vi "aggregator - v - real - interp.vi"(8 "number":dbl, 10 "init?":bool, 11 "requested size":i32=20) -> (0 "slope":dbl, 1 "interp average":dbl, 2 "mean":dbl, 3 "Array":dbl[](array[numeric]))   [LabVIEW 2018]
uses:
  agregator -- action.ctl
  linear interpolation - real.vi
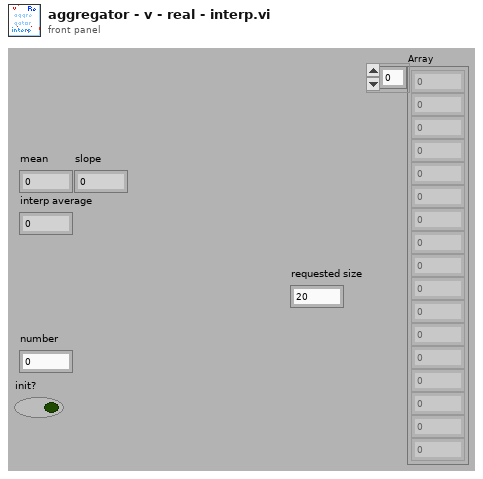
[diagram p1: front panel]
types:
  T1 = typedef "agregator -- action.ctl" = enum16{"append", "interpolate", "empty!", "force", "init", "scale", "read last"}
  T2 = typedef "interpolation state - real.ctl" = cluster{"requested size":i32, "Array":dbl[], "actual number of elements":i32}
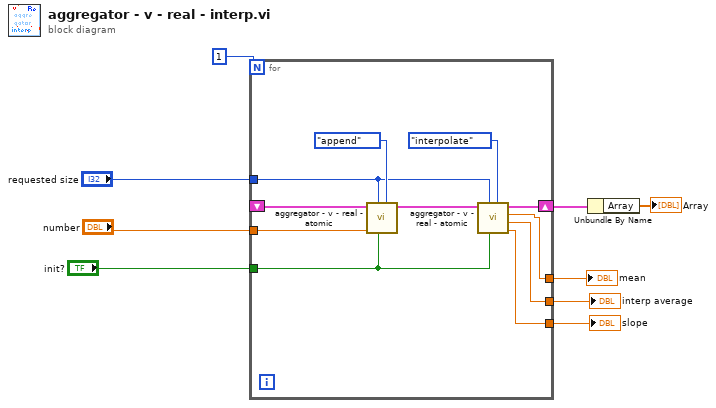
[diagram p0: block diagram]
diagram:
  n1 = for {
    N: 1 -> [_]
    tunnel: "requested size" -> [w11]
    tunnel: "number" -> [w20]
    tunnel: "init?" -> [w10]
    shift-right: [w15] -> w5
    shift-left: _ -> [w19]
    tunnel: [w14] -> w3
    tunnel: [w13] -> w2
    tunnel: [w12] -> w1
    n2 = call "aggregator - v - real - atomic.vi"("aggregator action"=agregator_--_action."append", "init?"=w10, "requested size"=w11, "number"=w20, "state IN"=w19) -> ("state OUT"=w16:T2)  [unwired: 3 in, 3 out]
    n3 = call "aggregator - v - real - atomic.vi"("aggregator action"=agregator_--_action."interpolate", "init?"=w10, "requested size"=w11, "state IN"=w16) -> ("slope"=w12:dbl, "interp average"=w13:dbl, "mean"=w14:dbl, "state OUT"=w15:T2)  [unwired: 4 in]
  }
  "mean" <- w3
  "interp average" <- w2
  "slope" <- w1
  n4 = Unbundle By Name(w5) -> ("Array"=→"Array":dbl[])
